vi "Item_OnPopupMenu.vi"(11 "Item Ref":T1) -> ()   [LabVIEW 2020, in "FlexWorker_Provider.lvlib"]
uses:
  <resource>/Framework/Providers/API/ItemRef.ctl
  <resource>/Framework/Providers/API/mxLvMenuItem.ctl
  FlexWorker_Provider.lvlib
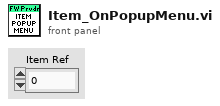
[diagram p1: front panel]
types:
  T1 = typedef "ItemRef.ctl" = u64
  T2 = typedef "mxLvMenuItem.ctl" = cluster{"Menu Name":string, "Description":string, "Icon File Name":path, "Menu Tag":string, "Enabled":bool, "Checked":bool, "Separator":bool, "Batchable":bool, "Weight":i32, "Batch Mode (Ignored if Not Batchable)":enum32{"Show If All Items Support Command", "Show If Any Items Support Command"}, "Menu Location":enum32{"<None>", "Project", "Project / Build Specifications", "Tools", "Tools / Source Control", "Tools / Real-Time Module", "Help"}, "Exclude From Getting Started Window Menu":bool}
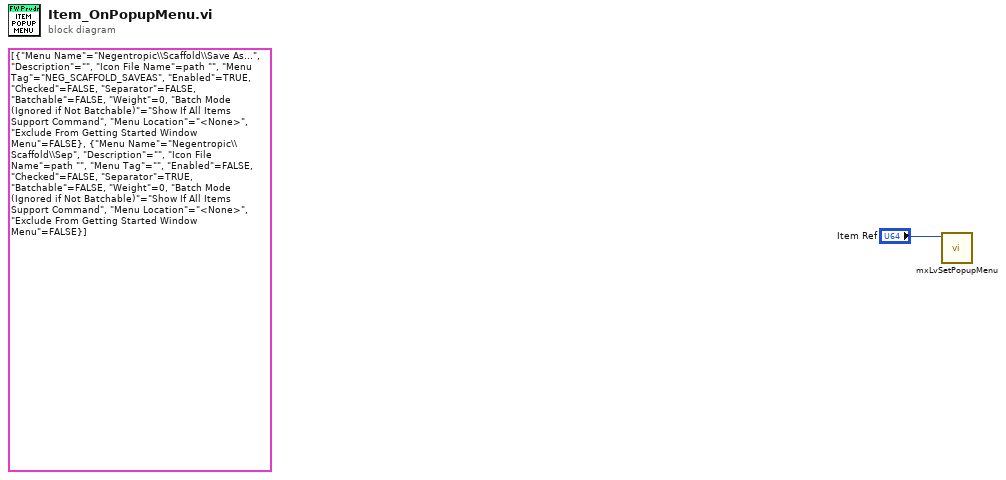
[diagram p0: block diagram]
diagram:
  (unwired) T2[] [{"Menu Name"="Negentropic\\Scaffold\\Save As...", "Description"="", "Icon File Name"=path "", "Menu Tag"="NEG_SCAFFOLD_SAVEAS", "Enabled"=TRUE, "Checked"=FALSE, "Separator"=FALSE, "Batchable"=FALSE, "Weight"=0, "Batch Mode (Ignored if Not Batchable)"=enum."Show If All Items Support Command", "Menu Location"=enum."<None>", "Exclude From Getting Started Window Menu"=FALSE}, {"Menu Name"="Negentropic\\Scaffold\\Sep", "Description"="", "Icon File Name"=path "", "Menu Tag"="", "Enabled"=FALSE, "Checked"=FALSE, "Separator"=TRUE, "Batchable"=FALSE, "Weight"=0, "Batch Mode (Ignored if Not Batchable)"=enum."Show If All Items Support Command", "Menu Location"=enum."<None>", "Exclude From Getting Started Window Menu"=FALSE}] ("Popup Menu Items")
  n1 = call <resource>:"mxLvSetPopupMenu.vi"("Item"="Item Ref") -> ()  [unwired: 9 in, 2 out]
